vi "make list.vi"() -> ()   [LabVIEW 2009]
panel:
  in  "Tab Control":enum32{"numeric", "numeric text"}(tab)=enum."numeric text"
  in  "start":i32
  in  "end":i32
  in  "delimiter (new line)":string="\n"
  in  "unformat string":string="%d"
  in  "copy to clipboard":bool=TRUE
  out "output":string
  in  "format string":string="<img src=\"images/%03d.png\">"
  in  "delimiter (Tab)":string="\t"
  # "Clipboard is source"
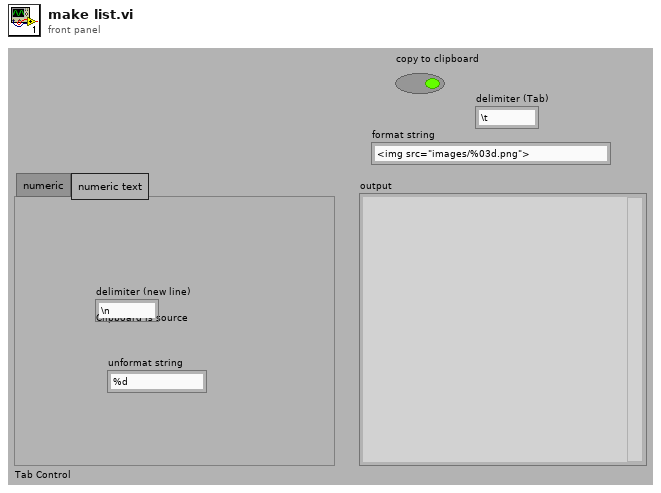
[diagram p1: front panel]
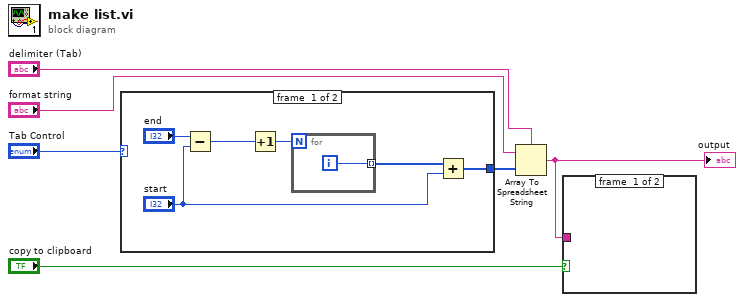
[diagram p0: block diagram]
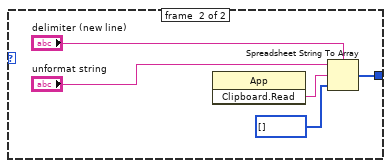
[diagram p2: hidden frame]
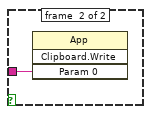
[diagram p3: hidden frame]
diagram:
  n1 = case shown="\"numeric text\"" "Tab Control" {
    tunnel: [w7 w14] -> w6
    frame #0 {
      n2 = Subtract(x="end", y="start") -> (x-y=w11:i32)
      n3 = Increment(x=w11) -> (x+1=w10:i32)
      n4 = for {
        N: w10 -> [_]
        tunnel: [w13] -> w9 mode=indexing
        i -> [w13]
      }
      n5 = Add(x=w9, y="start") -> (x+y=w7:i32[])
    }
    frame #1 {
      n6 = invoke class="App" method="Clipboard.Read"() -> ("Read Clipbrd"=w18:string)  [unwired: 3 in, 2 out]
      n7 = Spreadsheet String To Array(delimiter (Tab)="delimiter (new line)", format string="unformat string", spreadsheet string=w18, array type (2D Dbl)=i32[] []) -> (array=w14:i32[])
    }
  }
  n8 = Array To Spreadsheet String(delimiter (Tab)="delimiter (Tab)", array=w6, 3:"format string") -> (spreadsheet string=w2:string)
  "output" <- w2
  n9 = case shown="True" "copy to clipboard" {
    tunnel: w2 -> [_ w19]
    frame #0 {
    }
    frame #1 {
      n10 = invoke class="App" method="Clipboard.Write"("Param 0"=w19) -> ()  [unwired: 3 in, 4 out]
    }
  }
